vi "Notify SizeChange.vi"(8 "error in (no error)":errorcluster, 9 "Promise in":refnum<class "Promise.lvclass">, 10 "content size":T1) -> (0 "error out":errorcluster)   [LabVIEW 2021, in "TipStripOOPanel.lvlib" / "TipPanel.lvclass"]
uses:
  TipPanel.lvclass
  <vilib>/Utility/miscctls.llb/LVBoundsTypeDef.ctl
  <vilib>/Futures/Futures/Promise/Promise.lvclass
  TipPanel.lvclass/TipPanel.ctl
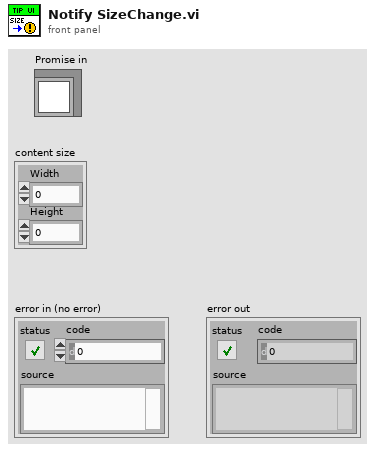
[diagram p1: front panel]
types:
  T1 = typedef "LVBoundsTypeDef.ctl" = cluster{"Width":u32, "Height":u32}
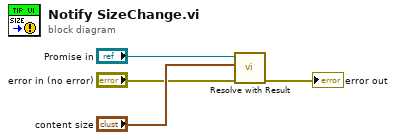
[diagram p0: block diagram]
diagram:
  n1 = call <vilib>:"Resolve with Result.vi"("error in (no error)"="error in (no error)", "Result"="content size", "Promise in"="Promise in") -> ("error out"=→"error out":errorcluster)  [unwired: 8 in]
